vi "CRYTree Navigate.vi"(7 "Tags":refnum<vi>, 10 "Start Tag In":string, 11 "Tree In":refnum<vi>) -> (3 "Tree Out":refnum<vi>)   [LabVIEW 2013]
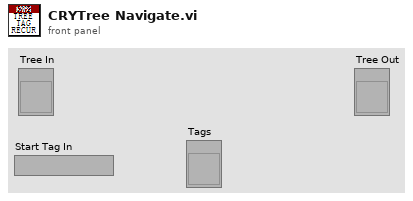
[diagram p1: front panel]
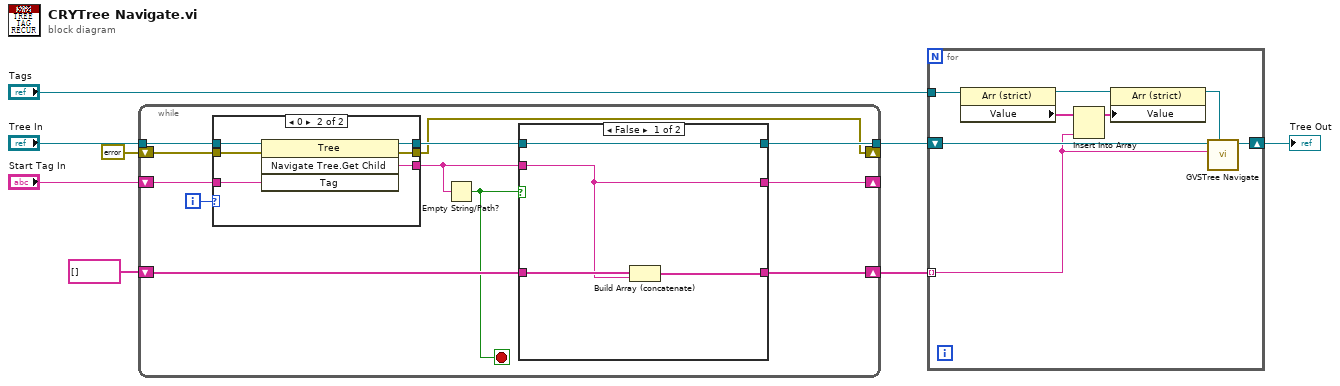
[diagram p0: block diagram]
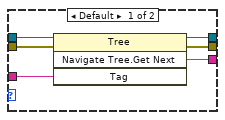
[diagram p3: hidden frame]
diagram:
  n1 = while {
    tunnel: "Tree In" -> [w20]
    shift-right: [w13] -> _
    shift-left: "Start Tag In" -> [w9]
    shift-right: [w11] -> _
    shift-left: errorcluster {"status"=FALSE, "code"=0, "source"=""} ("error out") -> [w19]
    shift-right: [w17] -> w7
    shift-left: string[] [] -> [w18]
    tunnel: [w15] -> w6
    i -> [w10]
    stop <- w12 stop-if-true
    n2 = case shown="0" w10 {
      tunnel: w20 -> [w33 w39]
      tunnel: w9 -> [w32 w38]
      tunnel: [w30 w37] -> w14
      tunnel: w19 -> [w31 w36]
      tunnel: [w29 w35] -> w11
      tunnel: [w28 w34] -> w16
      frame Default {
        n3 = invoke class="Tree" method="Navigate Tree.Get Next"(reference=w33, error in=w31, "Tag"=w32) -> (reference out=w28:refnum<vi>, error out=w29:errorcluster, "Navigate Tree:Get Next Item"=w30:string)  [unwired: 1 in, 1 out]
      }
      frame 0 {
        n4 = invoke class="Tree" method="Navigate Tree.Get Child"(reference=w39, error in=w36, "Tag"=w38) -> (reference out=w34:refnum<vi>, error out=w35:errorcluster, "Navigate Tree:Get Child"=w37:string)  [unwired: 1 in, 1 out]
      }
    }
    n5 = Empty String/Path?(string/path=w14) -> (empty?=w12:bool)
    n6 = case shown="False" w12 {
      tunnel: w18 -> [w23 w27]
      tunnel: [w22 w27] -> w17
      tunnel: w16 -> [w24 w25]
      tunnel: [w24 w25] -> w15
      tunnel: w14 -> [w21 w26]
      tunnel: [w21 w26] -> w13
      frame False {
        n7 = Build Array (concatenate)(w23, w21) -> (w22:string[])
      }
      frame True {
      }
    }
  }
  n8 = for {
    tunnel: w7 -> [w46] mode=indexing
    tunnel: "Tags" -> [w45]
    shift-right: [w40] -> w2
    shift-left: w6 -> [w47]
    n9 = property class="Arr (strict)"(reference=w45) -> (reference out=w44:refnum<vi>, "Value"=w41:string[])  [unwired: 1 in, 1 out]
    n10 = Insert Into Array(array=w41, new element=w46) -> (w43:string[])  [unwired: 1 in]
    n11 = property class="Arr (strict)"(reference=w44, "Value"=w43) -> (reference out=w42:refnum<vi>)  [unwired: 1 in, 1 out]
    n12 = call "GVSTree Navigate.vi"("Tags"=w42, "Start Tag In"=w46, "Tree In"=w47) -> ("Tree Out"=w40:refnum<vi>)  [unwired: 8 in]
  }
  "Tree Out" <- w2
